vi "Check for Existing Handler.vi"(8 "error in (no error)":errorcluster, 11 "ExecAnchor in":refnum<class "ExecAnchor.lvclass">) -> (0 "error out":errorcluster, 2 "Existing Handler":bool, 3 "ExecAnchor out":refnum<class "ExecAnchor.lvclass">)   [LabVIEW 2020, in "ExecAnchor.lvclass"]
uses:
  ExecAnchor.lvclass
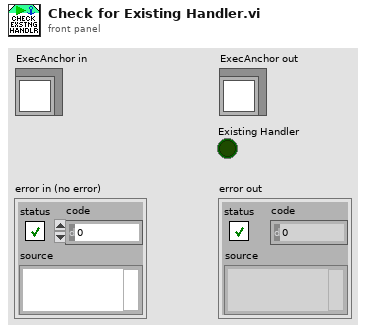
[diagram p1: front panel]
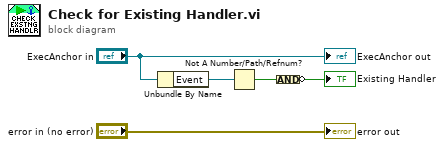
[diagram p0: block diagram]
diagram:
  n1 = Unbundle By Name("ExecAnchor in") -> ("Event"=w4:refnum<user-event>)
  n2 = Not A Number/Path/Refnum?(number/path/refnum=w4) -> (NaN/Path/Refnum?=w3:bool)
  n3 = Compound Arithmetic op=AND(w3) -> (invert →"Existing Handler":bool)
  "error out" <- "error in (no error)"
  "ExecAnchor out" <- "ExecAnchor in"
